vi "Host Main.vi"() -> ()   [LabVIEW 2013]
doc: "This application launches and executes the Tag Bus Data framework configuration for the specified target alias. This is a simple example of the framework API functions, but may also be a suitable starting point for a Host UI or Thick Client that is running a local version of the framework."
uses:
  <vilib>/NI/Module Execution Interface/Engine Runtime/Execution States.ctl
  <vilib>/NI/Module Execution Interface/Engine Runtime/Fault.ctl
  <vilib>/NI/Tag Bus Module Framework/runtime/error classification.ctl
  <vilib>/NI/Module Execution Interface/Engine Runtime/Engine Runtime Interface.lvclass
  <vilib>/NI/Current Value Table/DataTypes/Single_Read.vi
  <vilib>/NI/Current Value Table/DataTypes/Single_Write.vi
  <vilib>/NI/Current Value Table/Type to Enum.vi
  <vilib>/NI/Current Value Table/DataTypes/Single_Type To Enum.vi
  <vilib>/NI/Current Value Table/FGVs/CVT Globals.vi
  <vilib>/NI/Current Value Table/FGVs/Tag Memory.vi
  <vilib>/NI/Current Value Table/Memory Block.vi
  <vilib>/NI/Current Value Table/DataTypes/Single_Memory Block.vi
  <vilib>/NI/DCAF/Tag Editor Core/Framework Configuration Classes/target runtime/PL_Target Runtime.lvclass
  <vilib>/NI/Current Value Table/Current Value Table.lvlib
  <vilib>/NI/Tag Bus Module Framework/runtime/TBM module execution interface.lvclass
panel:
  in  "Write":sgl
  out "Read":sgl
  in  "configuration file path":path=path "c:/TestConfig.pcfg"
  in  "target alias":string="PXI"
  out "engine status":T4(array[cluster])
  in  "stop":bool
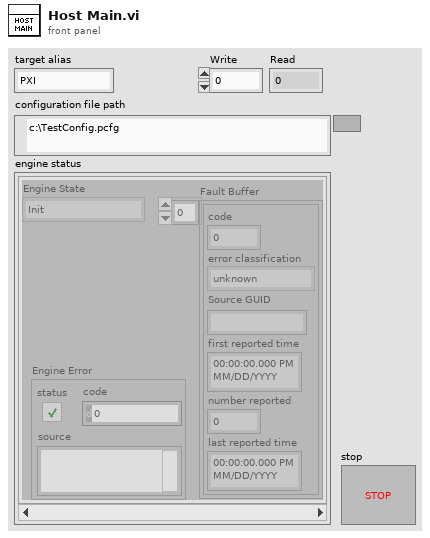
[diagram p1: front panel]
types:
  T1 = typedef "Engine Runtime Interface.lvclass/Execution States.ctl" = enum16{"Init", "Pre-Operational", "Safe-Operational", "Operational", "Stopped"}
  T2 = typedef "Engine Runtime Interface.lvclass/Fault.ctl" = cluster{"code":i32, "error classification":T3, "Source GUID":string, "first reported time":timestamp, "number reported":u32, "last reported time":timestamp}
  T3 = typedef "TBM module execution interface.lvclass/error classification.ctl" = enum16{"unknown", "none", "trivial", "recoverable", "critical"}
  T4 = cluster{"Engine State":T1, "Fault Buffer":T2[], "Engine Error":errorcluster}[]
  T5 = cluster{"Engine State":T1, "faults":T2[], "Engine Error":errorcluster}
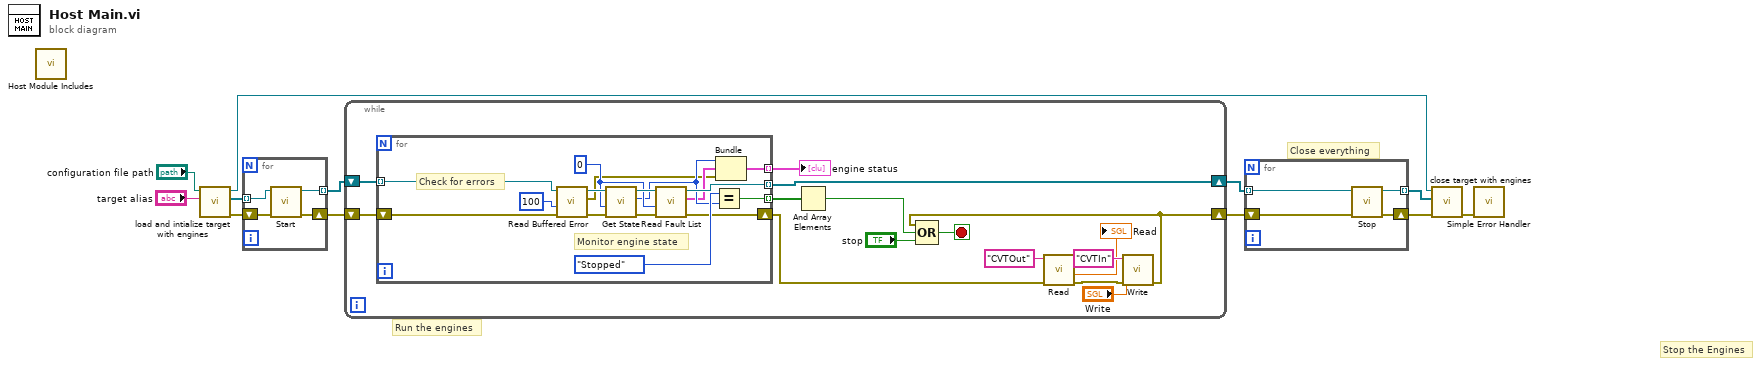
[diagram p0: block diagram]
diagram:
  # "Close everything"
  # "Stop the Engines"
  # "Run the engines"
  n1 = call "Host Module Includes.vi"() -> ()  [unwired: 12 in]
  n2 = call <vilib>:"load and intialize target with engines.vi"("target alias"="target alias", "file path"="configuration file path") -> ("error out"=w9:errorcluster, "engine runtime interfaces"=w8:refnum<class "Engine Runtime Interface.lvclass">[], "target runtime"=w5:refnum<class "PL_Target Runtime.lvclass">)  [unwired: 7 in]
  n3 = for {
    tunnel: [w16] -> w12 mode=indexing
    tunnel: w8 -> [w13] mode=indexing
    shift-right: [w15] -> w2
    shift-left: w9 -> [w14]
    n4 = call-dynamic "Start.vi"("error in"=w14, "Engine Runtime Interface in"=w13) -> ("error out"=w15:errorcluster, "Engine Runtime Interface out"=w16:refnum<class "Engine Runtime Interface.lvclass">)  [unwired: 8 in]
  }
  n5 = while {
    shift-right: [w29] -> w11
    shift-left: w12 -> [w31]
    shift-right: [w17] -> w10
    shift-left: w2 -> [w30]
    stop <- w27 stop-if-true
    n6 = for {
      tunnel: w31 -> [w47] mode=indexing
      tunnel: [w38] -> w29 mode=indexing
      tunnel: [w42] -> w25 mode=indexing
      shift-right: [w37] -> w19
      shift-left: w30 -> [w46]
      tunnel: [w32] -> w26 mode=indexing
      w36 = 0 ("timeout (-1)")
      # "Monitor engine state"
      # "Check for errors"
      n7 = call-dynamic "Read Buffered Error.vi"("error in"=w46, "timeout in ms (0)"=100, "Engine Runtime Interface in"=w47) -> ("error out"=w44:errorcluster, "Engine Error"=w33:errorcluster, "Engine Runtime Interface out"=w45:refnum<class "Engine Runtime Interface.lvclass">)  [unwired: 6 in]
      n8 = call-dynamic "Get State.vi"("error in"=w44, "timeout (-1)"=w36, "Engine Runtime Interface in"=w45) -> ("error out"=w40:errorcluster, "Engine State"=w35:T1, "Engine Runtime Interface out"=w39:refnum<class "Engine Runtime Interface.lvclass">)  [unwired: 6 in]
      n9 = call-dynamic "Read Fault List.vi"("error in"=w40, "timeout (-1)"=w36, "Engine Runtime Interface in"=w39) -> ("error out"=w37:errorcluster, "faults"=w34:T2[], "Engine Runtime Interface out"=w38:refnum<class "Engine Runtime Interface.lvclass">)  [unwired: 6 in]
      n10 = Equal?(x=Execution_States."Stopped" ("Engine State"), y=w35) -> (x = y?=w42:bool)
      n11 = Bundle("Engine State"=w35, "faults"=w34, "Engine Error"=w33) -> (w32:T5)  [unwired: 1 in]
    }
    "engine status" <- w26
    n12 = And Array Elements(Boolean array=w25) -> (logical AND=w24:bool)
    n13 = call-poly <vilib>:"Read.vi"("error in (no error)"=w19, "Tag Name"="CVTOut") -> ("error out"=w18:errorcluster, "Value"=→"Read":sgl)  [unwired: 8 in]
    n14 = call-poly <vilib>:"Write.vi"("error in (no error)"=w18, "Value"="Write", "Tag Name"="CVTIn") -> ("error out"=w17:errorcluster)  [unwired: 8 in]
    n15 = Compound Arithmetic op=OR(w17, w24, "stop") -> (w27:bool)
  }
  n16 = for {
    tunnel: w11 -> [w51] mode=indexing
    shift-right: [w48] -> w4
    shift-left: w10 -> [w50]
    tunnel: [w49] -> w6 mode=indexing
    n17 = call-dynamic "Stop.vi"("error in"=w50, "Engine Runtime Interface in"=w51) -> ("error out"=w48:errorcluster, "Engine Runtime Interface out"=w49:refnum<class "Engine Runtime Interface.lvclass">)  [unwired: 8 in]
  }
  n18 = call <vilib>:"close target with engines.vi"("error in"=w4, "Engine Runtime Interfaces"=w6, "Target Runtime"=w5) -> ("error out"=w1:errorcluster)  [unwired: 8 in]
  n19 = call <vilib>:"Simple Error Handler.vi"("error in (no error)"=w1) -> ()  [unwired: 4 in, 5 out]
